vi "Check for Uncommitted Files.vi"(8 "error in":errorcluster, 11 "Peer Review in":refnum<class "Peer Review.lvclass">) -> (0 "error out":errorcluster, 3 "Peer Review out":refnum<class "Peer Review.lvclass">)   [LabVIEW 2020, in "Peer Review.lvclass"]
uses:
  Peer Review.lvclass
  Peer Review.lvclass/Peer Review.ctl
  TypeDefs/Commit Info.ctl
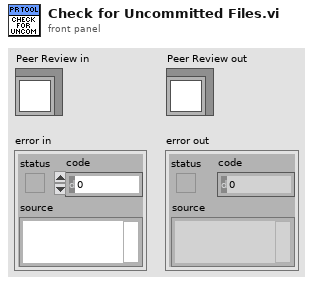
[diagram p1: front panel]
types:
  T1 = typedef "Peer Review.lvclass/Commit Info.ctl" = cluster{"Commit ID":i32, "Hash":string, "Merge Commit?":bool, "Merge Hash":string, "Author":string, "Time Stamp":timestamp, "Description":string, "File Count":i32, "File List":string[]}
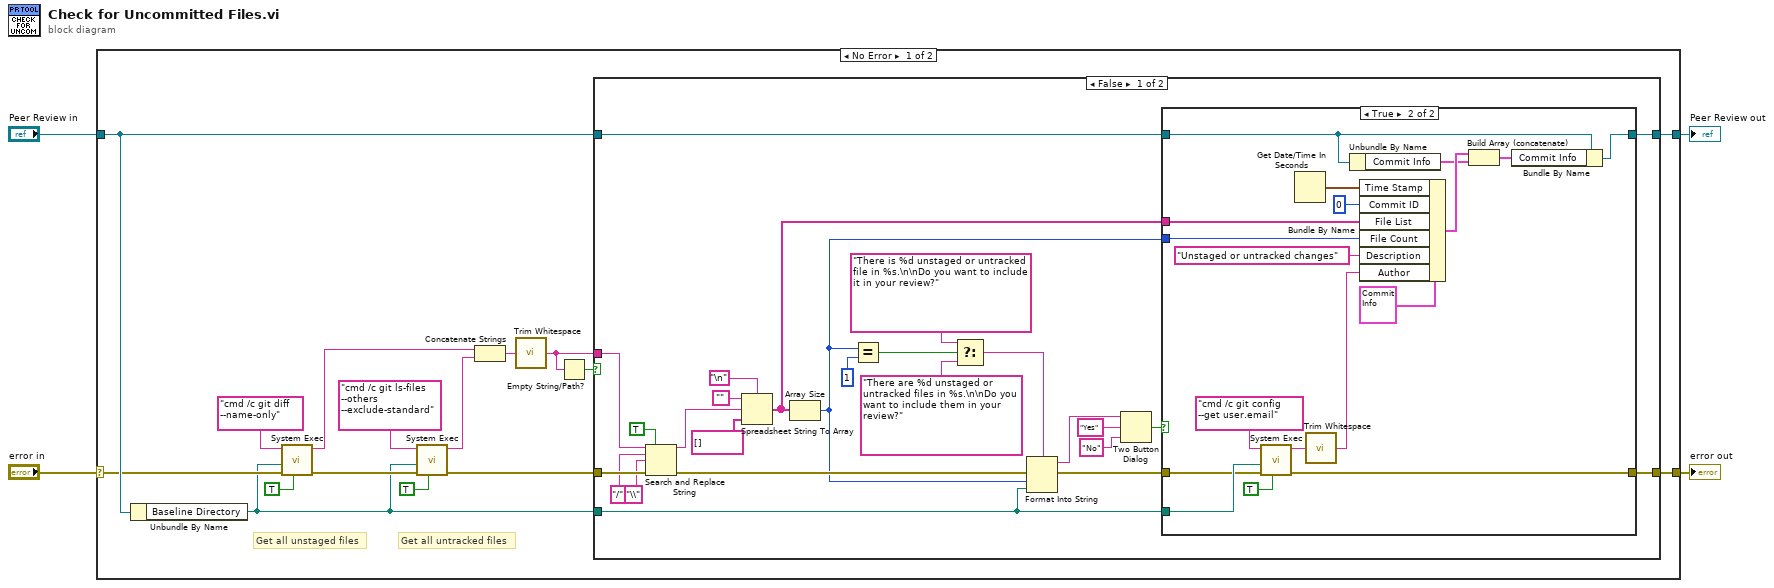
[diagram p0: block diagram]
diagram:
  n1 = case shown="No Error" "error in" {
    selector: "error in" -> [w14 w70]
    tunnel: [w19 w70] -> w3
    tunnel: [w18 w69] -> w1
    tunnel: "Peer Review in" -> [w17 w69]
    frame No Error {
      # "Get all untracked files"
      # "Get all unstaged files"
      n2 = Unbundle By Name(w17) -> ("Baseline Directory"=w5:path)
      n3 = call <vilib>:"System Exec.vi"("run minimized? (F)"=TRUE, "error in (no error)"=w14, "working directory"=w5, "command line"="cmd /c git diff --name-only") -> ("error out"=w10:errorcluster, "standard output"=w7:string)  [unwired: 4 in, 2 out]
      n4 = call <vilib>:"System Exec.vi"("run minimized? (F)"=TRUE, "error in (no error)"=w10, "working directory"=w5, "command line"="cmd /c git ls-files --others --exclude-standard") -> ("error out"=w9:errorcluster, "standard output"=w8:string)  [unwired: 4 in, 2 out]
      n5 = Concatenate Strings(w7, w8) -> (w11:string)
      n6 = call <vilib>:"Trim Whitespace.vi"("string"=w11) -> ("trimmed string"=w6:string)  [unwired: 1 in]
      n7 = Empty String/Path?(string/path=w6) -> (empty?=w16:bool)
      n8 = case shown="False" w16 {
        tunnel: w6 -> [w34 _]
        tunnel: w9 -> [w39 w67]
        tunnel: [w43 w67] -> w19
        tunnel: w5 -> [w24 _]
        tunnel: [w41 w68] -> w18
        tunnel: w17 -> [w40 w68]
        frame False {
          n9 = Search and Replace String(replace all?=TRUE ("replace all? (F)"), input string=w34, search string="/", replace string="\\" ("replace string (\"\")"), error in=w39) -> (result string=w38:string, error out=w25:errorcluster)  [unwired: 3 in, 2 out]
          n10 = Spreadsheet String To Array(delimiter (Tab)="\n", format string="", spreadsheet string=w38, array type (2D Dbl)=string[] []) -> (array=w42:string[])
          n11 = Array Size(array=w42) -> (size(s)=w22:i32)
          n12 = Equal?(x=w22, y=1) -> (x = y?=w31:bool)
          n13 = Select(t="There is %d unstaged or untracked file in %s.\n\nDo you want to include it in your review?" ("message"), s=w31, f="There are %d unstaged or untracked files in %s.\n\nDo you want to include them in your review?" ("message")) -> (s? t:f=w32:string)
          n14 = Format Into String(format string=w32, error in=w25, w22, w24) -> (resulting string=w33:string, error out=w23:errorcluster)  [unwired: 1 in]
          n15 = Two Button Dialog(message=w33, 1:"No" ("F button name (\"Cancel\")"), 2:"Yes" ("T button name (\"OK\")")) -> (T button?=w21:bool)
          n16 = case shown="True" w21 {
            tunnel: [w47 w62] -> w43
            tunnel: w42 -> [_ w61]
            tunnel: [w48 w56] -> w41
            tunnel: w40 -> [w48 w54]
            tunnel: w24 -> [_ w51]
            tunnel: w23 -> [w47 w50]
            tunnel: w22 -> [_ w49]
            frame False {
              # "Don't include unstaged or untracked files."
            }
            frame True {
              n17 = call <vilib>:"System Exec.vi"("run minimized? (F)"=TRUE, "error in (no error)"=w50, "working directory"=w51, "command line"="cmd /c git config --get user.email") -> ("error out"=w62:errorcluster, "standard output"=w55:string)  [unwired: 4 in, 2 out]
              n18 = Get Date/Time In Seconds() -> (seconds since 1Jan1904=w60:timestamp)
              n19 = call <vilib>:"Trim Whitespace.vi"("string"=w55) -> ("trimmed string"=w52:string)  [unwired: 1 in]
              n20 = Unbundle By Name(w54) -> ("Commit Info"=w53:T1[])
              n21 = Bundle By Name(cluster=T1 {"Commit ID"=0, "Hash"="", "Merge Commit?"=FALSE, "Merge Hash"="", "Author"="", "Time Stamp"=timestamp(0 s since 1904-01-01), "Description"="", "File Count"=0, "File List"=[]}, "Time Stamp"=w60, "Commit ID"=0, "File List"=w61, "File Count"=w49, "Description"="Unstaged or untracked changes", "Author"=w52) -> (w58:T1)
              n22 = Build Array (concatenate)(w58, w53) -> (w57:T1[])
              n23 = Bundle By Name(cluster=w54, "Commit Info"=w57) -> (w56:refnum<class "Peer Review.lvclass">)
            }
          }
        }
        frame True {
          # "No unstaged or untracked files, so do nothing."
        }
      }
    }
    frame Error {
    }
  }
  "error out" <- w3
  "Peer Review out" <- w1
